vi "Test New Recompose.vi"() -> ()   [LabVIEW 2026, in "VILab.lvlib"]
uses:
  VILab.lvlib
  SubVIs/Decompose VI (Refnum).vi
  <userlib>/_OpenG.lib/array/array.llb/Filter 1D Array with Scalar (Boolean)__ogtk.vi
  <userlib>/_OpenG.lib/array/array.llb/openg_array.lvlib
panel:
  out "filtered item indices 2":i32[](array[numeric])
  out "filtered item indices":i32[](array[numeric])
  out "Block Diagram XML":string
  out "Front Panel XML":string
  out "Rebuilt BD XML":string
  out "Rebuilt FP XML":string
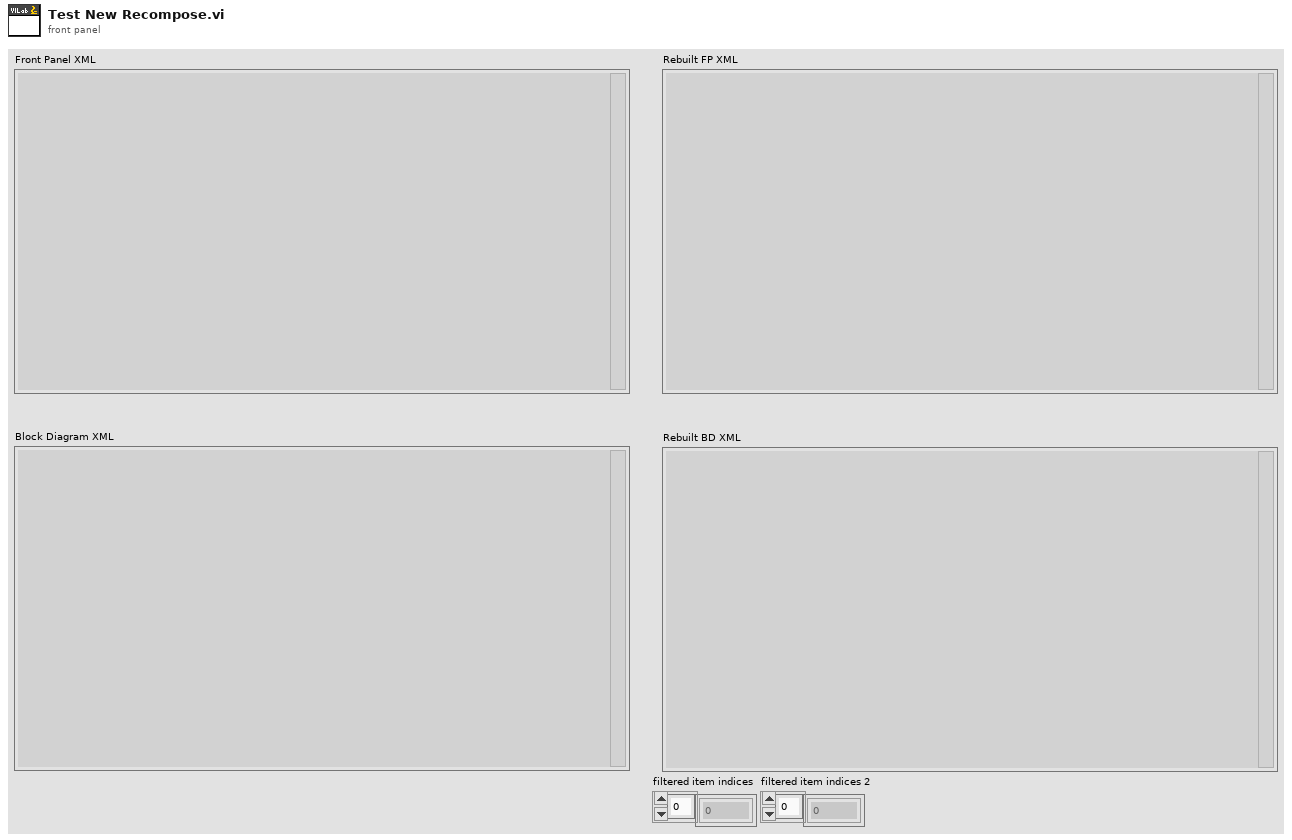
[diagram p1: front panel]
types:
  T1 = typedef "VILab.lvlib/Resource.ctl" = cluster{"type":u32, "id":i32, "name":string, "binary data":string}
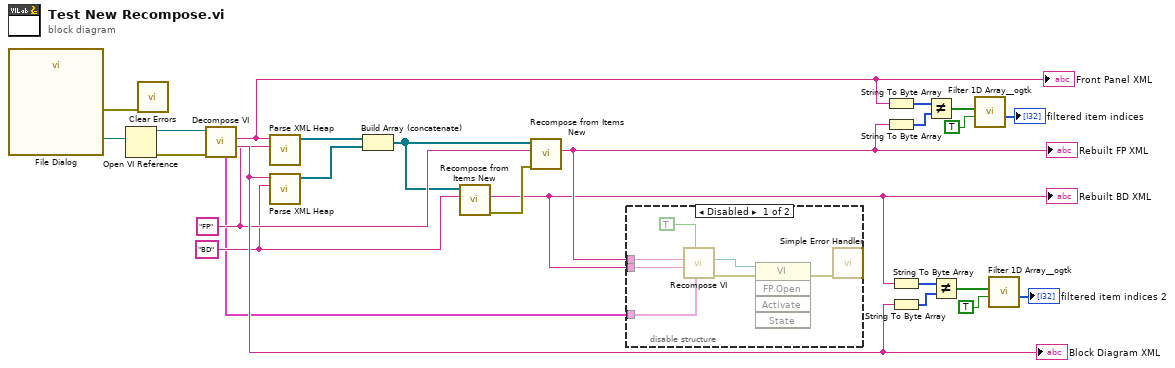
[diagram p0: block diagram]
diagram:
  w6 = "BD" ("Root Parent")
  w7 = "FP" ("Root Parent")
  n1 = call "File Dialog"() -> ("selected path"=w23:path, "error out"=w22:errorcluster)  [unwired: 12 in, 2 out]
  n2 = Open VI Reference(vi path=w23) -> (vi reference=w25:refnum<vi>, error out=w24:errorcluster)  [unwired: 5 in]
  n3 = call <vilib>:"Clear Errors.vi"("error in (no error)"=w22) -> ()  [unwired: 5 in, 2 out]
  n4 = call-poly "Decompose VI.vi"("error in (no error)"=w24, "VI Ref"=w25) -> ("Block Diagram XML"=w10:string, "Front Panel XML"=w11:string, "Other resources"=w2:T1[])  [unwired: 5 in, 2 out]
  "Front Panel XML" <- w11
  "Block Diagram XML" <- w10
  n5 = call "Parse XML Heap.vi"("Root Parent"=w7, "XML"=w11) -> ("Items"=w9:refnum<class "Data Item.lvclass">[])  [unwired: 8 in, 1 out]
  n6 = call "Parse XML Heap.vi"("Root Parent"=w6, "XML"=w10) -> ("Items"=w8:refnum<class "Data Item.lvclass">[])  [unwired: 8 in, 1 out]
  n7 = Build Array (concatenate)(w9, w8) -> (w1:refnum<class "Data Item.lvclass">[])
  n8 = call "Recompose from Items New.vi"("Tree Tag"=w6, "All Data"=w1) -> ("error out"=w5:errorcluster, "XML String"=w3:string)  [unwired: 8 in]
  "Rebuilt BD XML" <- w3
  n9 = call "Recompose from Items New.vi"("error in (no error)"=w5, "Tree Tag"=w7, "All Data"=w1) -> ("XML String"=w4:string)  [unwired: 7 in, 1 out]
  "Rebuilt FP XML" <- w4
  n10 = disable-structure shown="Disabled" {
    disable-tunnel: w4 -> [w32 _]
    disable-tunnel: w3 -> [w31 _]
    disable-tunnel: w2 -> [w29 _]
    frame Disabled {
      n11 = call "Recompose VI.vi"("Other resources (default)"=w29, "Open VI? (F)"=TRUE, "Block Diagram XML"=w31, "Front Panel XML"=w32) -> ("error out"=w28:errorcluster, "VI Refnum (if opened)"=w26:refnum<vi>)  [unwired: 5 in, 1 out]
      n12 = invoke class="VI" method="FP.Open"(reference=w26, error in=w28) -> (error out=w27:errorcluster)  [unwired: 3 in, 4 out]
      n13 = call <vilib>:"Simple Error Handler.vi"("error in (no error)"=w27) -> ()  [unwired: 4 in, 5 out]
    }
    frame Enabled {
    }
  }
  n14 = String To Byte Array(string=w11) -> (unsigned byte array=w21:u8[])
  n15 = String To Byte Array(string=w4) -> (unsigned byte array=w20:u8[])
  n16 = String To Byte Array(string=w3) -> (unsigned byte array=w19:u8[])
  n17 = String To Byte Array(string=w10) -> (unsigned byte array=w18:u8[])
  n18 = Not Equal?(x=w21, y=w20) -> (x != y?=w17:bool[])
  n19 = Not Equal?(x=w19, y=w18) -> (x != y?=w12:bool[])
  n20 = call-poly <userlib>:"Filter 1D Array__ogtk.vi"("items to filter"=TRUE, "array"=w17) -> ("filtered item indices"=→"filtered item indices":i32[])  [unwired: 4 in, 1 out]
  n21 = call-poly <userlib>:"Filter 1D Array__ogtk.vi"("items to filter"=TRUE, "array"=w12) -> ("filtered item indices"=→"filtered item indices 2":i32[])  [unwired: 4 in, 1 out]
